vi "Text Timestamp String.vi"(1 "Seconds":dbl) -> (0 "Timestamp String":string)   [LabVIEW 2010]
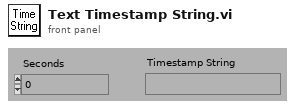
[diagram p1: front panel]
types:
  T1 = cluster{"second":i32, "minute":i32, "hour":i32, "day of month":i32, "month":i32, "year":i32, "day of week":i32, "day of year":i32, "is DST":i32}
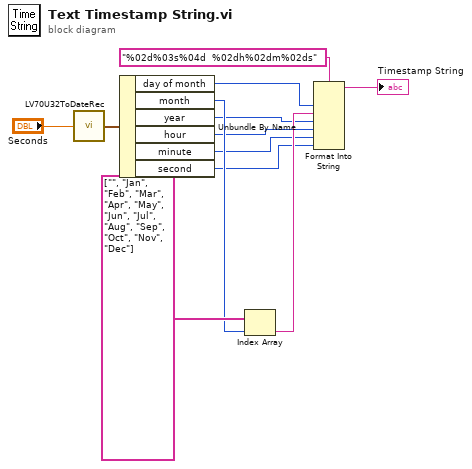
[diagram p0: block diagram]
diagram:
  n1 = call <vilib>:"LV70U32ToDateRec.vi"("Time"="Seconds") -> ("date time rec"=w12:T1)
  n2 = Unbundle By Name(w12) -> ("day of month"=w8:i32, "month"=w9:i32, "year"=w6:i32, "hour"=w5:i32, "minute"=w4:i32, "second"=w3:i32)
  n3 = Index Array(array=string[] ["", "Jan", "Feb", "Mar", "Apr", "May", "Jun", "Jul", "Aug", "Sep", "Oct", "Nov", "Dec"], index=w9) -> (element=w7:string)
  n4 = Format Into String(format string="%02d%03s%04d  %02dh%02dm%02ds", w8, w7, w6, w5, w4, w3) -> (resulting string=→"Timestamp String":string)  [unwired: 2 in, 1 out]
